vi "CrawlingPrechargeState.vi"(8 "error in (no error)":errorcluster, 9 "Cluster in":T2, 10 "Enum in":T1, 11 "Actual Start [i]":i64) -> (0 "error out":errorcluster, 2 "Cluster out":T2, 3 "Enum":T1)   [LabVIEW 2018]
uses:
  Type_Def Actuator Controls.ctl
  Type_Def_Current_state_output.ctl
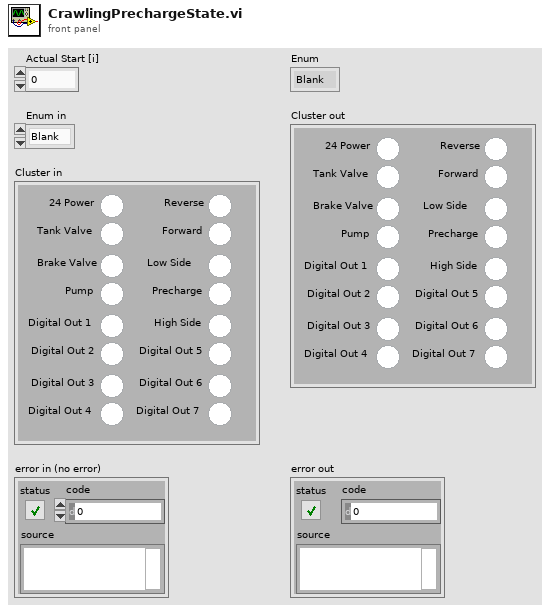
[diagram p1: front panel]
types:
  T1 = typedef "Type_Def_Current_state_output.ctl" = enum16{"Blank", "Systems Check", "Idle", "Ready", "Pushing", "CrawlingPrecharge", "Braking", "Fault", "Boot Up", "Unpowered", "Crawling", "Shutdown", "Service Push", "Service Wait", "Vent", "Precharge", "Cooldown"}
  T2 = typedef "Type_Def Actuator Controls.ctl" = cluster{"Reverse ":bool, "Forward":bool, "Low Side":bool, "Precharge":bool, "High Side":bool, "Digital Out 5":bool, "Digital Out 6":bool, "Digital Out 7 ":bool, "24 Power":bool, "Tank Valve ":bool, "Brake Valve":bool, "Pump":bool, "Digital Out 1 ":bool, "Digital Out 2":bool, "Digital Out 3":bool, "Digital Out 4 ":bool}
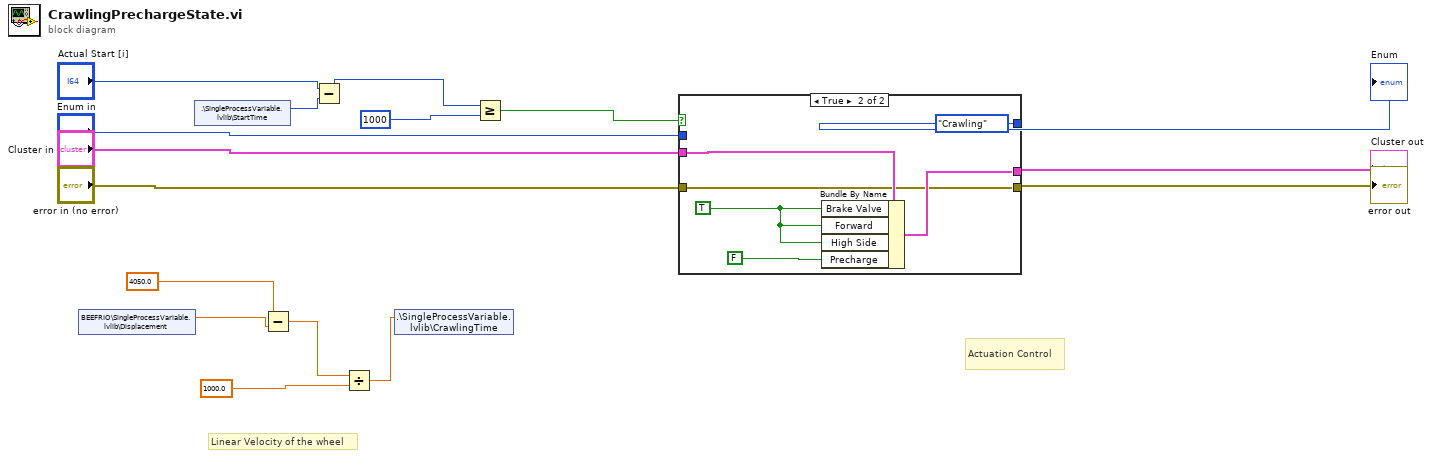
[diagram p0: block diagram]
diagram:
  # "Linear Velocity of the wheel"
  # "Actuation Control"
  n1 = shared-variable "BEEFRIO\\SingleProcessVariable.lvlib\\Displacement"() -> (w13:dbl)  [unwired: 1 in, 1 out]
  n2 = shared-variable ".\\SingleProcessVariable.lvlib\\StartTime"() -> (w7:i64)  [unwired: 1 in, 1 out]
  n3 = Subtract(x=4050.0, y=w13) -> (x-y=w14:dbl)
  n4 = Subtract(x="Actual Start [i]", y=w7) -> (x-y=w9:i64)
  n5 = Divide(x=w14, y=1000.0) -> (x/y=w16:dbl)
  n6 = shared-variable ".\\SingleProcessVariable.lvlib\\CrawlingTime"(w16) -> ()  [unwired: 1 in, 1 out]
  n7 = Greater Or Equal?(x=w9, y=i64 1000) -> (x >= y?=w11:bool)
  n8 = case shown="True" w11 {
    tunnel: "Enum in" -> [w19 _]
    tunnel: [w19 Type_Def_Current_state_output."Crawling"] -> w2
    tunnel: "Cluster in" -> [w18 w24]
    tunnel: [w18 w23] -> w4
    tunnel: [w17 w22] -> w5
    tunnel: "error in (no error)" -> [w17 w22]
    frame False {
    }
    frame True {
      w21 = TRUE ("Digital Out 5")
      n9 = Bundle By Name(cluster=w24, "Brake Valve"=w21, "Forward"=w21, "High Side"=w21, "Precharge"=FALSE ("Digital Out 5")) -> (w23:T2)
    }
  }
  "error out" <- w5
  "Cluster out" <- w4
  "Enum" <- w2
